vi "ex1.vi"() -> ()   [LabVIEW 2021]
panel:
  out "x/y":dbl
  out "x*y":dbl
  out "x-y":dbl
  out "x+y":dbl
  in  "Y":dbl
  in  "X":dbl
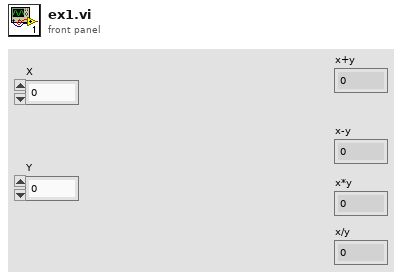
[diagram p1: front panel]
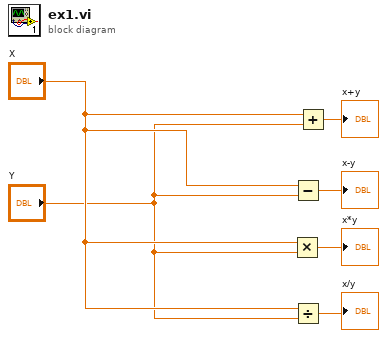
[diagram p0: block diagram]
diagram:
  n1 = Multiply(x="X", y="Y") -> (x*y=→"x*y":dbl)
  n2 = Subtract(x="X", y="Y") -> (x-y=→"x-y":dbl)
  n3 = Divide(x="X", y="Y") -> (x/y=→"x/y":dbl)
  n4 = Add(x="X", y="Y") -> (x+y=→"x+y":dbl)
